vi "onCreated.vi"(8 "error in (no error)":errorcluster, 11 "PM":refnum<class "OPM.lvclass">) -> (0 "error out":errorcluster, 3 "PM out":refnum<class "OPM.lvclass">)   [LabVIEW 2017, in "OPM.lvclass"]
doc: "JKI State Machine Objects (SMO) 1.3.0.56\nJKI - JKI\nCopyright (c) 2017, JKI"
uses:
  OPM.lvclass
  D:/Program Files (x86)/National Instruments/LabVIEW 2017/vi.lib/JKI/JKI SMO/SMO/SMO.lvclass
  D:/upwork/Laser Measurement Tool/Laser/project/Subsystems/MeasuringDevice/MeasuringDevice.lvclass
  Typedefs/Configuration--Cluster.ctl
  CircularBuffer/types/type.DBL/type.DBL.lvclass
  D:/upwork/Laser Measurement Tool/Laser/project/Subsystems/CircularBuffer/types/type/type.lvclass
  MeasuringDevice/MeasuringDevice.lvclass
  <vilib>/Utility/config.llb/NI_LVConfig.lvlib
  CircularBuffer/CircularBuffer.lvclass
  <vilib>/JKI/JKI SMO/SMO/SMO.lvclass
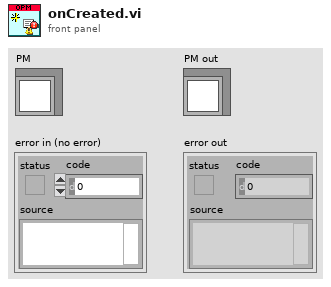
[diagram p1: front panel]
types:
  T1 = typedef "OPM.lvclass/Configuration--Cluster.ctl" = cluster{"VISA Resource":string}
  T2 = typedef "NI_LVConfig.lvlib/Config Data RefNum.ctl" = refnum<k1>
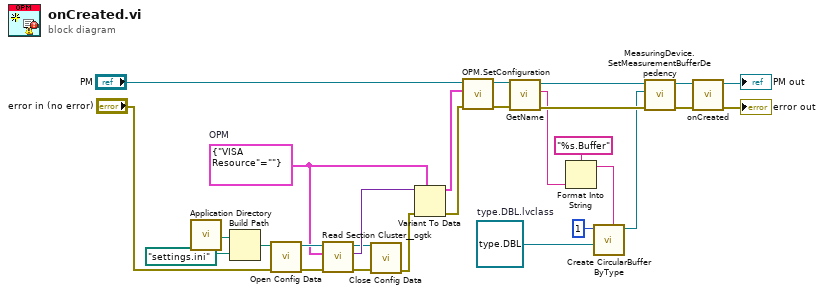
[diagram p0: block diagram]
diagram:
  w18 = refnum<class "type.DBL.lvclass"> refnum  # type.DBL.lvclass
  w22 = T1 {"VISA Resource"=""}  # OPM
  n1 = call <vilib>:"Application Directory.vi"() -> ("Application Directory"=w26:path)
  n2 = Build Path(base path=w26, name or relative path=path "settings.ini") -> (appended path=w28:path)
  n3 = call <vilib>:"Open Config Data.vi"("error in (no error)"="error in (no error)", "configuration file path"=w28) -> ("error out"=w23:errorcluster, "refnum"=w25:T2)  [unwired: 7 in, 1 out]
  n4 = call <userlib>:"Read Section Cluster__ogtk.vi"("error in (no error)"=w23, "Section Formatted Cluster Type"=w22, "refnum"=w25) -> ("error out"=w3:errorcluster, "Section Formatted Cluster"=w24:variant, "dup refnum"=w2:T2)  [unwired: 4 in, 2 out]
  n5 = call <vilib>:"Close Config Data.vi"("error in (no error)"=w3, "refnum"=w2) -> ("error out"=w1:errorcluster)  [unwired: 8 in, 1 out]
  n6 = Variant To Data(error in=w1, type=w22, Variant=w24) -> (data=w21:T1, error out=w4:errorcluster)
  n7 = call "OPM.SetConfiguration.vi"("error in (no error)"=w4, "Configuration"=w21, "PM"="PM") -> ("error out"=w10:errorcluster, "PM out"=w11:refnum<class "OPM.lvclass">)  [unwired: 7 in]
  n8 = call <vilib>:"GetName.vi"("error in (no error)"=w10, "SMO"=w11) -> ("error out"=w16:errorcluster, "Name"=w12:string, "SMO out"=w17:refnum<class "OPM.lvclass">)  [unwired: 7 in]
  n9 = Format Into String(format string="%s.Buffer", w12) -> (resulting string=w13:string)  [unwired: 2 in, 1 out]
  n10 = call "Create CircularBuffer ByType.vi"("Buffer Name"=w13, "type"=w18, "BufferSize"=1) -> ("CircularBuffer out"=w15:refnum<class "CircularBuffer.lvclass">)  [unwired: 6 in, 2 out]
  n11 = call "MeasuringDevice.SetMeasurementBufferDepedency.vi"("error in (no error)"=w16, "CircularBuffer"=w15, "MeasuringDevice"=w17) -> ("error out"=w8:errorcluster, "MeasuringDevice"=w9:refnum<class "OPM.lvclass">)  [unwired: 7 in]
  n12 = call-parent "onCreated.vi"("error in (no error)"=w8, "SMO"=w9) -> ("error out"=→"error out":errorcluster, "SMO out"=→"PM out":refnum<class "OPM.lvclass">)  [unwired: 8 in]
